vi "Initialize.vi"(7 "Serial Configuration":T1={"Baud Rate"=9600, "Parity"=0, "Data Bits"=7, "Stop Bits"=10} {"Stop Bits" items=["1"=10, "2"=20]; "Data Bits" items=["7"=7, "8"=8]; "Parity" items=["None", "Odd", "Even"]; "Baud Rate" items=["300"=300, "600"=600, "1200"=1200, "2400"=2400, "4800"=4800, "9600"=9600, "19200"=19200]}, 8 "error in (no error)":errorcluster, 9 "Reset (True)":bool=TRUE, 10 "ID Query (True)":bool=TRUE, 11 "VISA resource name":refnum<visa-resource-name>) -> (0 "error out":errorcluster, 3 "VISA resource name out":refnum<visa-resource-name>)   [LabVIEW 2023, in "Fluke Molbox 1 Plus.lvlib"]
doc: "Establishes communication with the instrument and optionally performs an instrument identification query and/or an instrument reset. It also places the instrument in a default state needed for other instrument driver operations. Therefore, call this VI before calling other instrument driver VIs for this instrument. Generally, you need to call the Initialize VI only once at the beginning of an application."
uses:
  Fluke Molbox 1 Plus.lvlib
panel:
  # "(c) 2012 National Instruments.  ALL RIGHTS RESERVED."
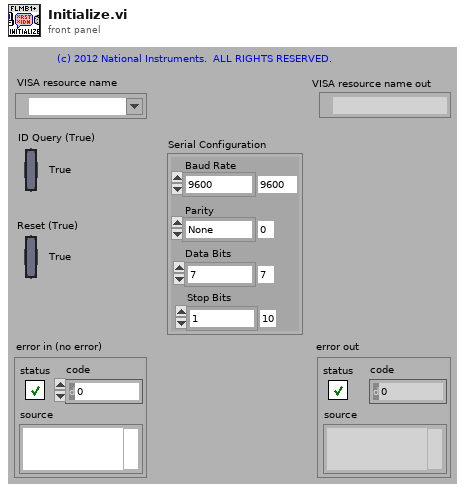
[diagram p1: front panel]
types:
  T1 = cluster{"Baud Rate":u32, "Parity":u16, "Data Bits":u16, "Stop Bits":u16}
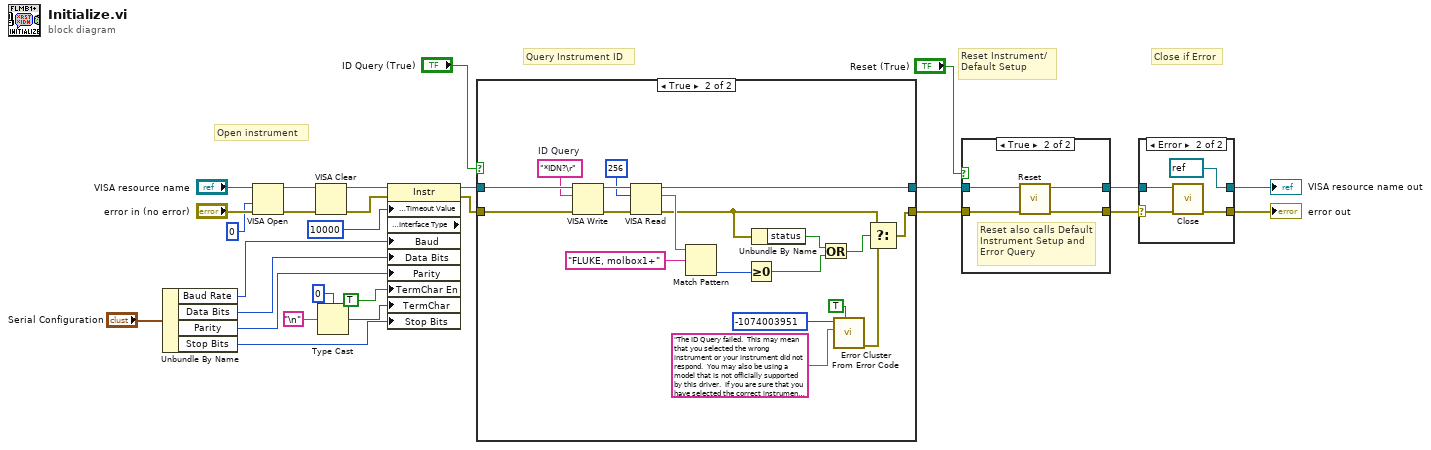
[diagram p0: block diagram]
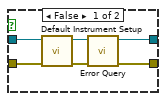
[diagram p3: hidden frame]
diagram:
  # "Close if Error"
  # "Query Instrument ID"
  # "Reset Instrument/\nDefault Setup"
  # "Open instrument"
  n1 = Unbundle By Name("Serial Configuration") -> ("Baud Rate"=w3:u32, "Data Bits"=w2:u16, "Parity"=w1:u16, "Stop Bits"=w4:u16)
  n2 = VISA Open(access mode=u32 0, error in (no error)="error in (no error)", VISA resource name="VISA resource name") -> (VISA resource name=w17:refnum<visa-resource-name>, error out=w16:errorcluster)  [unwired: 2 in]
  n3 = VISA Clear(VISA resource name=w17, error in (no error)=w16) -> (VISA resource name out=w15:refnum<visa-resource-name>, error out=w14:errorcluster)
  n4 = Type Cast(type=u8 0 ("Serial Settings:Baud Rate"), x="\n" ("Line Feed Constant")) -> (*(type *) &x=w7:u8)
  n5 = property on="Property Node" class="Instr" props=["General Settings:Timeout Value", "Interface Information:Interface Type", "Baud", "Data Bits", "Parity", "TermChar En", "TermChar", "Stop Bits"](reference=w15, error in=w14, "General Settings:Timeout Value"=u32 10000, "Baud"=w3, "Data Bits"=w2, "Parity"=w1, "TermChar En"=TRUE ("Message Based Settings:Termination Character Enable"), "TermChar"=w7, "Stop Bits"=w4) -> (reference out=w20:refnum<visa-resource-name>, error out=w19:errorcluster)  [unwired: 1 out]
  n6 = case shown="True" "ID Query (True)" {
    tunnel: [w28 w48] -> w26
    tunnel: [w29 w45] -> w27
    tunnel: w20 -> [w29 w46]
    tunnel: w19 -> [w28 w47]
    frame False {
    }
    frame True {
      w39 = "*IDN?\r"  # ID Query
      n7 = VISA Write(VISA resource name=w46, write buffer=w39, error in (no error)=w47) -> (VISA resource name out=w43:refnum<visa-resource-name>, error out=w42:errorcluster)  [unwired: 1 out]
      n8 = VISA Read(VISA resource name=w43, byte count=u32 256, error in (no error)=w42) -> (VISA resource name out=w45:refnum<visa-resource-name>, read buffer=w44:string, error out=w33:errorcluster)  [unwired: 1 out]
      n9 = Match Pattern(string=w44, regular expression="FLUKE, molbox1+") -> (offset past match=w34:i32)  [unwired: 1 in, 3 out]
      n10 = Greater Or Equal To 0?(x=w34) -> (x >= 0?=w31:bool)
      n11 = Unbundle By Name(w33) -> ("status"=w32:bool)
      n12 = Or(x=w32, y=w31) -> (x .or. y?=w30:bool)
      n13 = call <vilib>:"Error Cluster From Error Code.vi"("show call chain? (False)"=TRUE, "error message (\"\")"="The ID Query failed.  This may mean that you selected the wrong instrument or your instrument did not respond.  You may also be using a model that is not officially supported by this driver.  If you are sure that you have selected the correct instrument and it is responding, try disabling the ID Query." ("Source (VI Name)"), "error code (0)"=-1074003951 ("Code")) -> ("error out"=w38:errorcluster)  [unwired: 6 in]
      n14 = Select(t=w33, s=w30, f=w38) -> (s? t:f=w48:errorcluster)
    }
  }
  n15 = case shown="True" "Reset (True)" {
    tunnel: w26 -> [w53 w55]
    tunnel: [w50 w58] -> w10
    tunnel: w27 -> [w54 w56]
    tunnel: [w51 w57] -> w11
    frame False {
      n16 = call "Default Instrument Setup.vi"("error in (no error)"=w53, "VISA resource name"=w54) -> ("error out"=w49:errorcluster, "VISA resource name out"=w52:refnum<visa-resource-name>)  [unwired: 8 in]
      n17 = call "Error Query.vi"("error in (no error)"=w49, "VISA resource name"=w52) -> ("error out"=w50:errorcluster, "VISA resource name out"=w51:refnum<visa-resource-name>)  [unwired: 6 in, 2 out]
    }
    frame True {
      # "Reset also calls Default Instrument Setup and Error Query"
      n18 = call "Reset.vi"("error in (no error)"=w55, "VISA resource name"=w56) -> ("error out"=w58:errorcluster, "VISA resource name out"=w57:refnum<visa-resource-name>)  [unwired: 8 in]
    }
  }
  n19 = case shown="Error" w10 {
    selector: w10 -> [w59 w62]
    tunnel: w11 -> [w60 w63]
    tunnel: [w60 refnum<visa-resource-name> refnum ("VISA resource name out")] -> w13
    tunnel: [w59 w64] -> w12
    frame No Error {
    }
    frame Error {
      n20 = call "Close.vi"("error in (no error)"=w62, "VISA resource name"=w63) -> ("error out"=w64:errorcluster)  [unwired: 9 in]
    }
  }
  "VISA resource name out" <- w13
  "error out" <- w12
